vi "test_libssh2_session_init_ex (recv callback).vi"() -> ()   [LabVIEW 2013, in "libssh2_integration_tests.lvlib"]
uses:
  libssh2_integration_tests.lvlib
  libssh2/libssh2_session_abstract.ctl
  libssh2/libssh2_session_callback_type.ctl
  libssh2/libssh2_init_default.vi
  libssh2/libssh2_session_handshake_tcp.vi
  libssh2/libssh2.lvlib
  <vilib>/addons/_JKI Toolkits/Caraya/classes/Assert/Assert.lvclass
  <vilib>/addons/_JKI Toolkits/Caraya/classes/Test/Test.lvclass
panel:
  out "error out":errorcluster
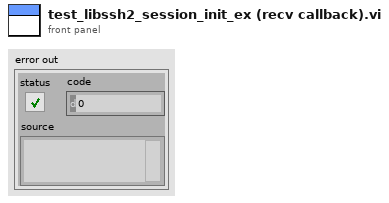
[diagram p1: front panel]
types:
  T1 = typedef "libssh2.lvlib/libssh2_session_abstract.ctl" = cluster{"send":refnum<vi>, "receive":refnum<vi>}
  T2 = typedef "libssh2.lvlib/libssh2_session_callback_type.ctl" = enum16{"Ignore", "Debug", "Disconnect", "MAC Error", "X11", "Send", "Receive", "Auth Agent", "Auth Agent Identities", "Auth Agent Sign"}
  T3 = typedef "libssh2.lvlib/Session Refnum.ctl" = refnum<k1>
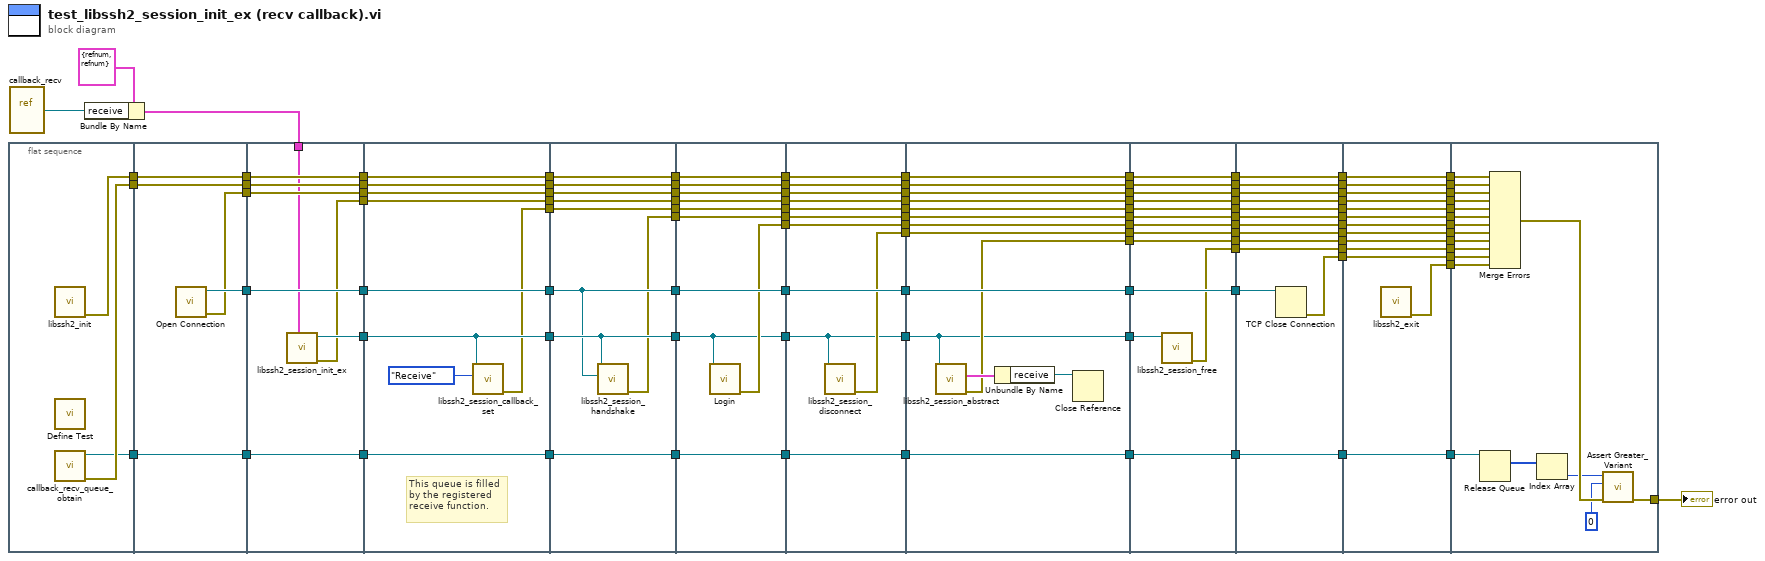
[diagram p0: block diagram]
diagram:
  n1 = flat-sequence {
    tunnel: [w109] -> w104
    tunnel: [w108] -> w87
    tunnel: [w107] -> w2
    tunnel: [w114] -> w103
    tunnel: w104 -> [w113]
    tunnel: [w113] -> w102
    tunnel: [w112] -> w101
    tunnel: w87 -> [w111]
    tunnel: [w111] -> w86
    tunnel: [w110] -> w3
    tunnel: w2 -> [w110]
    tunnel: w103 -> [w122]
    tunnel: [w122] -> w82
    tunnel: w102 -> [w121]
    tunnel: [w121] -> w80
    tunnel: w101 -> [w120]
    tunnel: [w120] -> w78
    tunnel: [w119] -> w76
    tunnel: [w118] -> w74
    tunnel: w86 -> [w117]
    tunnel: [w117] -> w72
    tunnel: w83 -> [w116]
    tunnel: [w115] -> w4
    tunnel: w3 -> [w115]
    tunnel: w82 -> [w131]
    tunnel: [w131] -> w81
    tunnel: w80 -> [w130]
    tunnel: [w130] -> w79
    tunnel: w78 -> [w129]
    tunnel: [w129] -> w77
    tunnel: w76 -> [w125]
    tunnel: [w125] -> w75
    tunnel: w74 -> [w128]
    tunnel: [w128] -> w73
    tunnel: w72 -> [w127]
    tunnel: [w127] -> w71
    tunnel: [w124] -> w70
    tunnel: [w123] -> w5
    tunnel: w4 -> [w123]
    tunnel: w81 -> [w136]
    tunnel: [w136] -> w67
    tunnel: w79 -> [w140]
    tunnel: [w140] -> w66
    tunnel: w77 -> [w139]
    tunnel: [w139] -> w65
    tunnel: [w138] -> w64
    tunnel: w75 -> [w138]
    tunnel: w73 -> [w137]
    tunnel: [w137] -> w63
    tunnel: [w135] -> w62
    tunnel: w71 -> [w134]
    tunnel: [w134] -> w61
    tunnel: w70 -> [w133]
    tunnel: [w133] -> w60
    tunnel: [w132] -> w6
    tunnel: w5 -> [w132]
    tunnel: w67 -> [w150]
    tunnel: [w150] -> w21
    tunnel: w66 -> [w149]
    tunnel: [w149] -> w20
    tunnel: w65 -> [w148]
    tunnel: [w148] -> w19
    tunnel: w64 -> [w142]
    tunnel: w63 -> [w147]
    tunnel: [w147] -> w18
    tunnel: w62 -> [w146]
    tunnel: [w146] -> w17
    tunnel: w61 -> [w145]
    tunnel: [w145] -> w16
    tunnel: w60 -> [w144]
    tunnel: [w144] -> w15
    tunnel: [w143] -> w14
    tunnel: [w142] -> w13
    tunnel: [w141] -> w7
    tunnel: w6 -> [w141]
    tunnel: w21 -> [w161]
    tunnel: [w161] -> w57
    tunnel: w20 -> [w160]
    tunnel: [w160] -> w56
    tunnel: w19 -> [w159]
    tunnel: [w159] -> w55
    tunnel: w18 -> [w158]
    tunnel: [w158] -> w54
    tunnel: [w157] -> w53
    tunnel: w17 -> [w156]
    tunnel: [w156] -> w52
    tunnel: w16 -> [w155]
    tunnel: [w155] -> w51
    tunnel: w15 -> [w154]
    tunnel: [w154] -> w50
    tunnel: w14 -> [w153]
    tunnel: [w153] -> w49
    tunnel: [w152] -> w48
    tunnel: w13 -> [w152]
    tunnel: [w151] -> w8
    tunnel: w7 -> [w151]
    tunnel: w57 -> [w175]
    tunnel: [w175] -> w45
    tunnel: w56 -> [w174]
    tunnel: [w174] -> w43
    tunnel: w55 -> [w173]
    tunnel: [w173] -> w41
    tunnel: w54 -> [w172]
    tunnel: [w172] -> w39
    tunnel: w53 -> [w171]
    tunnel: [w171] -> w37
    tunnel: w52 -> [w170]
    tunnel: [w170] -> w35
    tunnel: w51 -> [w169]
    tunnel: [w169] -> w33
    tunnel: w50 -> [w168]
    tunnel: [w168] -> w31
    tunnel: w49 -> [w167]
    tunnel: [w167] -> w29
    tunnel: w48 -> [w163]
    tunnel: [w164] -> w27
    tunnel: [w163] -> w25
    tunnel: [w162] -> w9
    tunnel: w8 -> [w162]
    tunnel: w45 -> [w188]
    tunnel: [w188] -> w44
    tunnel: w43 -> [w187]
    tunnel: [w187] -> w42
    tunnel: w41 -> [w186]
    tunnel: [w186] -> w40
    tunnel: w39 -> [w185]
    tunnel: [w185] -> w38
    tunnel: w37 -> [w184]
    tunnel: [w184] -> w36
    tunnel: w35 -> [w183]
    tunnel: [w183] -> w34
    tunnel: w33 -> [w182]
    tunnel: [w182] -> w32
    tunnel: w31 -> [w181]
    tunnel: [w181] -> w30
    tunnel: w29 -> [w180]
    tunnel: [w180] -> w28
    tunnel: w27 -> [w179]
    tunnel: [w179] -> w26
    tunnel: w25 -> [w178]
    tunnel: [w177] -> w22
    tunnel: [w176] -> w10
    tunnel: w9 -> [w176]
    tunnel: w44 -> [w201]
    tunnel: w42 -> [w200]
    tunnel: [w200] -> w100
    tunnel: w40 -> [w199]
    tunnel: [w199] -> w99
    tunnel: [w198] -> w98
    tunnel: w38 -> [w197]
    tunnel: [w197] -> w97
    tunnel: w36 -> [w196]
    tunnel: [w196] -> w96
    tunnel: w34 -> [w195]
    tunnel: [w195] -> w95
    tunnel: w32 -> [w194]
    tunnel: [w194] -> w85
    tunnel: w30 -> [w193]
    tunnel: [w193] -> w69
    tunnel: w28 -> [w192]
    tunnel: [w192] -> w59
    tunnel: w26 -> [w191]
    tunnel: [w191] -> w47
    tunnel: [w190] -> w23
    tunnel: w22 -> [w190]
    tunnel: [w189] -> w11
    tunnel: w10 -> [w189]
    tunnel: w100 -> [w214]
    tunnel: [w214] -> w94
    tunnel: w99 -> [w213]
    tunnel: [w213] -> w93
    tunnel: w98 -> [w212]
    tunnel: [w212] -> w92
    tunnel: [w211] -> w91
    tunnel: w97 -> [w210]
    tunnel: [w210] -> w90
    tunnel: w96 -> [w209]
    tunnel: [w209] -> w89
    tunnel: w95 -> [w208]
    tunnel: [w208] -> w88
    tunnel: w85 -> [w207]
    tunnel: [w207] -> w84
    tunnel: w69 -> [w206]
    tunnel: [w206] -> w68
    tunnel: w59 -> [w205]
    tunnel: [w205] -> w58
    tunnel: w47 -> [w204]
    tunnel: [w204] -> w46
    tunnel: [w203] -> w24
    tunnel: w23 -> [w203]
    tunnel: [w202] -> w12
    tunnel: w11 -> [w202]
    tunnel: w94 -> [w232]
    tunnel: w93 -> [w231]
    tunnel: w92 -> [w230]
    tunnel: w91 -> [w229]
    tunnel: w90 -> [w228]
    tunnel: w89 -> [w227]
    tunnel: [w225] -> w1
    tunnel: w88 -> [w224]
    tunnel: w84 -> [w223]
    tunnel: w68 -> [w222]
    tunnel: w58 -> [w221]
    tunnel: w46 -> [w220]
    tunnel: w24 -> [w219]
    tunnel: w12 -> [w217]
    frame #0 {
      n2 = call-poly "libssh2_init.vi"() -> ("error out"=w109:errorcluster)  [unwired: 11 in]
      n3 = call <vilib>:"Define Test.vi"() -> ()  [unwired: 10 in, 2 out]
      n4 = call "callback_recv_queue_obtain.vi"() -> ("error out"=w108:errorcluster, "queue out"=w107:refnum<queue>)  [unwired: 10 in]
    }
    frame #1 {
      n5 = call "Open Connection.vi"() -> ("error out"=w112:errorcluster, "connection ID"=w114:refnum<k5>)  [unwired: 10 in]
    }
    frame #2 {
      n6 = call "libssh2_session_init_ex.vi"("abstract"=w116) -> ("error out"=w118:errorcluster, "session"=w119:T3)  [unwired: 9 in]
    }
    frame #3 {
      # "This queue is filled\nby the registered\nreceive function."
      n7 = call "libssh2_session_callback_set.vi"("callback type"=libssh2_session_callback_type."Receive", "session"=w125) -> ("error out"=w124:errorcluster)  [unwired: 8 in, 1 out]
    }
    frame #4 {
      n8 = call-poly "libssh2_session_handshake.vi"("tcp connection"=w136, "session"=w138) -> ("error out"=w135:errorcluster)  [unwired: 9 in]
    }
    frame #5 {
      n9 = call "Login.vi"("session"=w142) -> ("error out"=w143:errorcluster)  [unwired: 10 in]
    }
    frame #6 {
      n10 = call "libssh2_session_disconnect.vi"("session"=w152) -> ("error out"=w157:errorcluster)  [unwired: 10 in]
    }
    frame #7 {
      n11 = call "libssh2_session_abstract.vi"("session"=w163) -> ("error out"=w164:errorcluster, "abstract"=w166:T1)  [unwired: 9 in]
      n12 = Unbundle By Name(w166) -> ("receive"=w165:refnum<vi>)
      n13 = Close Reference(reference=w165) -> ()  [unwired: 1 in, 1 out]
    }
    frame #8 {
      n14 = call "libssh2_session_free.vi"("session"=w178) -> ("error out"=w177:errorcluster)  [unwired: 10 in]
    }
    frame #9 {
      n15 = TCP Close Connection(connection ID=w201) -> (error out=w198:errorcluster)  [unwired: 2 in, 1 out]
    }
    frame #10 {
      n16 = call "libssh2_exit.vi"() -> ("error out"=w211:errorcluster)  [unwired: 11 in]
    }
    frame #11 {
      n17 = Release Queue(queue=w217) -> (remaining elements=w218:i32[])  [unwired: 2 in, 2 out]
      n18 = Merge Errors(w232, w223, w231, w228, w222, w224, w221, w227, w220, w219, w230, w229) -> (w226:errorcluster)
      n19 = Index Array(array=w218) -> (element=w216:i32)  [unwired: 1 in]
      n20 = call <vilib>:"Assert Greater_Variant.vi"("error in (no error)"=w226, "Y"=i64 0, "X"=w216) -> ("error out"=w225:errorcluster)  [unwired: 7 in, 1 out]
    }
  }
  n21 = vi-ref "callback_recv.vi"() -> (w105:refnum<vi>)
  n22 = Bundle By Name(cluster=T1 {"send"=refnum, "receive"=refnum} ("abstract"), "receive"=w105) -> (w83:T1)
  "error out" <- w1
